vi "KB-CalNew4Point.vi"(9 "矩形ROS 原始":string[](array[string]), 10 "Fitted Circle (Find Circular Edge 1) New":T3 {"Average SNR (dB)" format="%.2f"; "Average Strength" format="%.2f"; "Roundness (Real-World)" format="%.2f"; "Radius (Real-World)" format="%.2f"; "Center (Real-World)"."Y" format="%.2f"; "Center (Real-World)"."X" format="%.2f"; "Radius (Pixels)" format="%.2f"; "Center (Pixels)"."Y" format="%.2f"; "Center (Pixels)"."X" format="%.2f"}, 11 "原始寻心点":T2 {"Contours"."Type" items=["No Selection", "Point", "Line", "Rectangle", "Oval", "Polygon", "Freehand Region", "Annulus", "Unused2", "Unused3", "Broken Line", "Freehand Line", "Rotated Rectangle"]}) -> (3 "矩形ROS new":string[](array[string]))   [LabVIEW 2015]
panel:
  out "x":dbl
  out "x":dbl
  out "x+y 2":i32
  out "Picture Laser":T1(plugin-control)
  out "x+y":dbl
  out "y/2y/2":dbl
  out "x/2":dbl
  out "new bottom":dbl
  out "new Right":dbl
  out "new top":dbl
  out "new left":dbl
  out "Y 差值":dbl
  out "X 差值":dbl
  out "Y/2":dbl
  out "h":i32
  out "X/2":dbl
  out "w":i32
  out "Bottom":i32
  out "Right":i32
  out "TOP":i32
  out "Left":i32
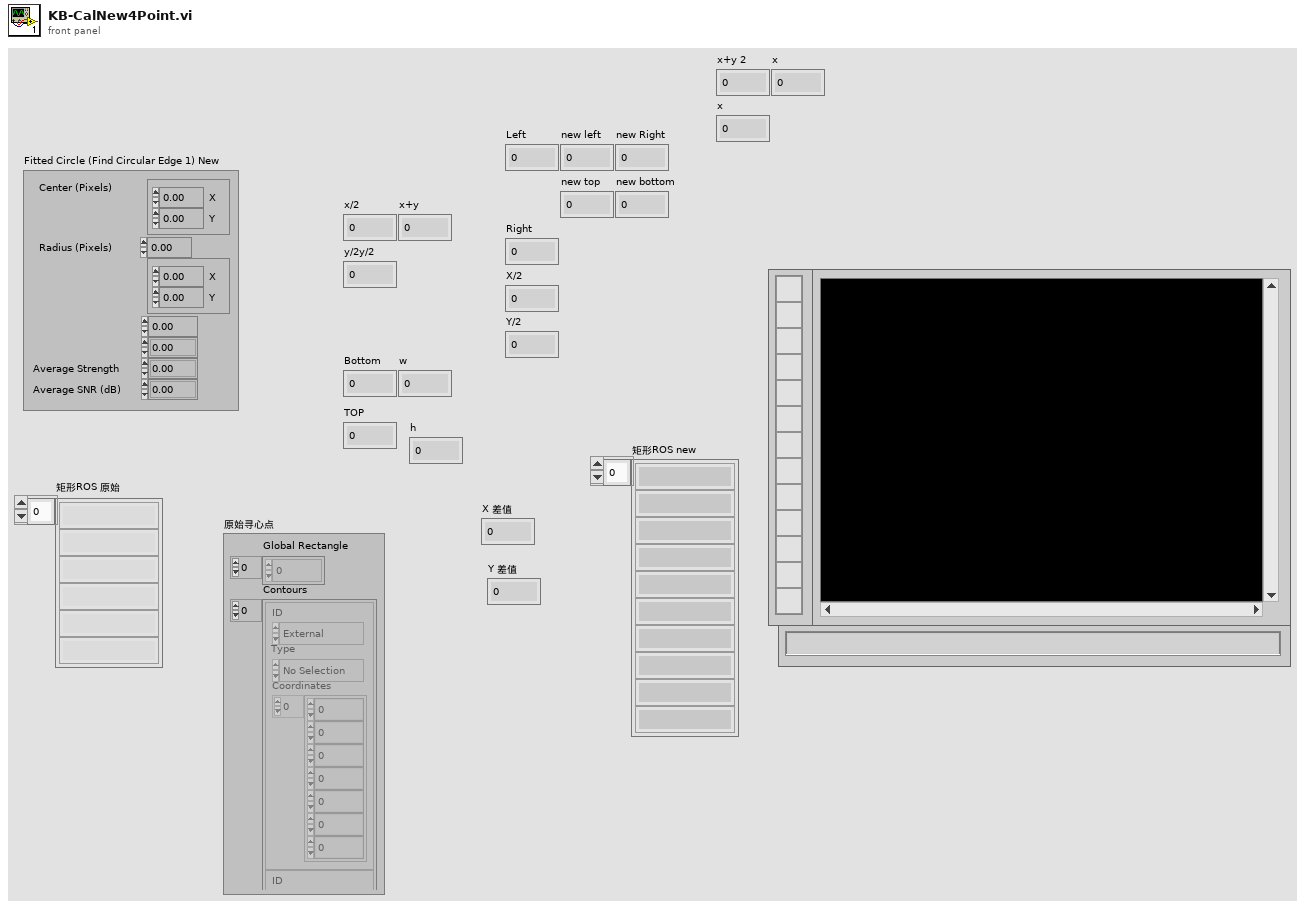
[diagram p1: front panel]
types:
  T1 = typedef "IMAQ Image.ctl" = refnum<image>
  T2 = typedef "ROI Descriptor" = cluster{"Global Rectangle":i32[], "Contours":cluster{"ID":enum32{"External", "Internal"}, "Type":u32, "Coordinates":i32[]}[]}
  T3 = cluster{"Center (Pixels)":cluster{"X":sgl, "Y":sgl}, "Radius (Pixels)":dbl, "Center (Real-World)":cluster{"X":sgl, "Y":sgl}, "Radius (Real-World)":dbl, "Roundness (Real-World)":dbl, "Average Strength":dbl, "Average SNR (dB)":dbl}
  T4 = cluster{"ID":enum32{"External", "Internal"}, "Type":u32, "Coordinates":i32[]}[]
  T5 = cluster{"ID":enum32{"External", "Internal"}, "Type":u32, "Coordinates":i32[]}
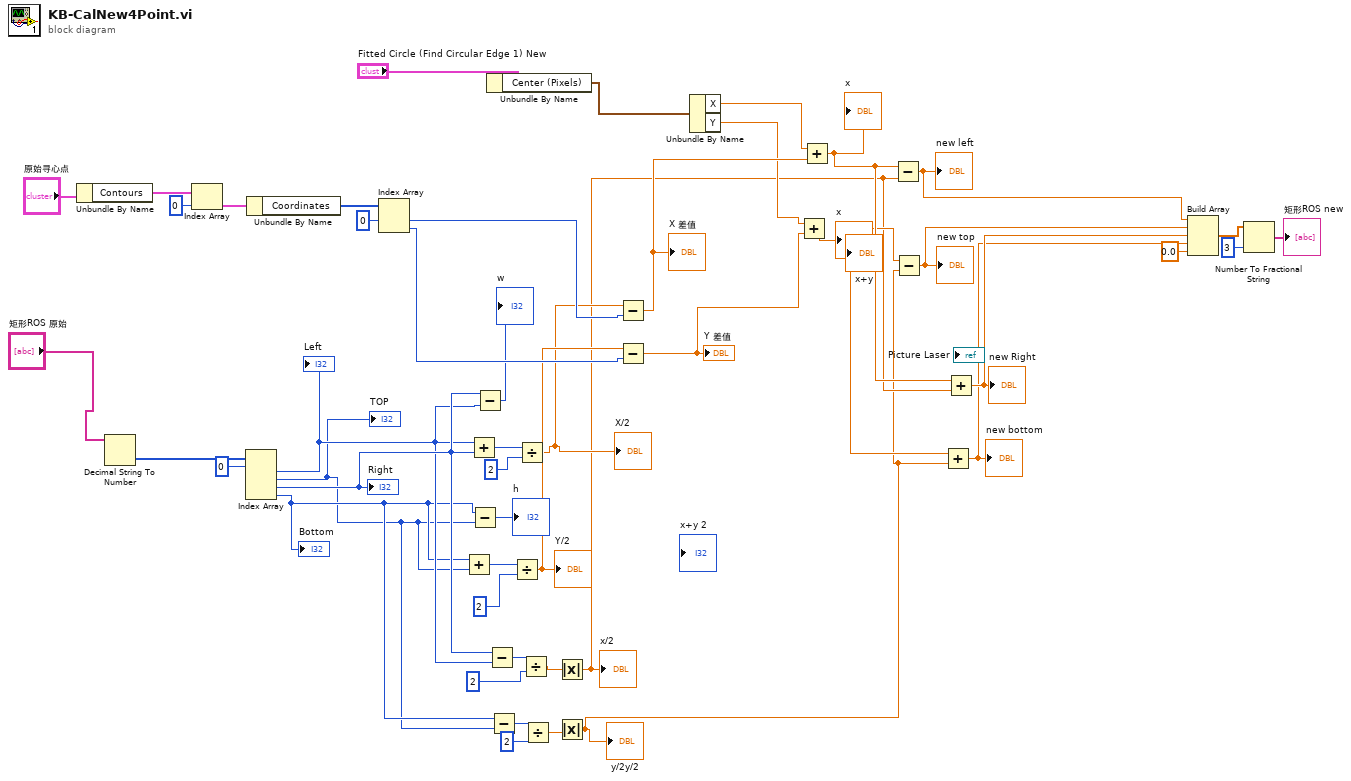
[diagram p0: block diagram]
diagram:
  n1 = Unbundle By Name("原始寻心点") -> ("Contours"=w42:T4)
  n2 = Decimal String To Number(string="矩形ROS 原始") -> (number=w45:i32[])  [unwired: 2 in, 1 out]
  n3 = Index Array(array=w42, index=0 ("索引")) -> (element=w40:T5)
  n4 = Index Array(array=w45, index #1=0 ("索引")) -> (element #1=w14:i32, element #2=w4:i32, element #3=w15:i32, element #4=w8:i32)  [unwired: 3 in]
  "Left" <- w14
  "TOP" <- w4
  "Right" <- w15
  "Bottom" <- w8
  n5 = Unbundle By Name(w40) -> ("Coordinates"=w39:i32[])
  n6 = Index Array(array=w39, index #1=0 ("索引")) -> (element #1=w37:i32, element #2=w36:i32)  [unwired: 1 in]
  n7 = Add(x=w8, y=w4) -> (x+y=w3:i32)
  n8 = Add(x=w14, y=w15) -> (x+y=w1:i32)
  n9 = Subtract(x=w8, y=w4) -> (x-y=→"h":i32)
  n10 = Subtract(x=w15, y=w14) -> (x-y=→"w":i32)
  n11 = Unbundle By Name("Fitted Circle (Find Circular Edge 1) New") -> ("Center (Pixels)"=w34:cluster{"X":sgl, "Y":sgl})
  n12 = Subtract(x=w15, y=w14) -> (x-y=w13:i32)
  n13 = Subtract(x=w8, y=w4) -> (x-y=w9:i32)
  n14 = Divide(x=w3, y=2 ("元素")) -> (x/y=w27:dbl)
  "Y/2" <- w27
  n15 = Divide(x=w1, y=2 ("元素")) -> (x/y=w16:dbl)
  "X/2" <- w16
  n16 = Divide(x=w13, y=2) -> (x/y=w11:dbl)
  n17 = Divide(x=w9, y=2) -> (x/y=w7:dbl)
  n18 = Absolute Value(x=w11) -> (abs(x)=w6:dbl)
  "x/2" <- w6
  n19 = Absolute Value(x=w7) -> (abs(x)=w5:dbl)
  "y/2y/2" <- w5
  n20 = Subtract(x=w16, y=w37) -> (x-y=w32:dbl)
  "X 差值" <- w32
  n21 = Subtract(x=w27, y=w36) -> (x-y=w30:dbl)
  "Y 差值" <- w30
  n22 = Unbundle By Name(w34) -> ("X"=w33:sgl, "Y"=w31:sgl)
  n23 = Add(x=w31, y=w30) -> (x+y=w28:dbl)
  "x+y" <- w28
  "x" <- w28
  n24 = Add(x=w33, y=w32) -> (x+y=w29:dbl)
  "x" <- w29
  n25 = Subtract(x=w29, y=w6) -> (x-y=w26:dbl)
  "new left" <- w26
  n26 = Subtract(x=w28, y=w5) -> (x-y=w25:dbl)
  "new top" <- w25
  n27 = Add(x=w28, y=w5) -> (x+y=w23:dbl)
  "new bottom" <- w23
  n28 = Add(x=w29, y=w6) -> (x+y=w24:dbl)
  "new Right" <- w24
  n29 = Build Array(w26, w25, w24, w23, 0.0 ("元素")) -> (w21:dbl[])
  n30 = Number To Fractional String(number=w21, precision (6)=i16 3 ("精度(6)")) -> (F-format string=→"矩形ROS new":string[])  [unwired: 2 in]
